vi "Intensity Check.vi"() -> ()   [LabVIEW 2020]
uses:
  <vilib>/Instr/_visa.llb/VISA Configure Serial Port (Instr).vi
panel:
  out "x+1":dbl
  in  "Take signal?":bool
  in  "Step Angle":dbl=10.0 format="%#_13g"
  in  "½Ð¤Å«ö¥ª¤W¨¤ªº°±¤îµ{¦¡":bool
  in  "iXon exposure time (sec)":dbl=0.15
  out "Currently Angle : (Analyzer)  2":string
  out "?":dbl(knob) scale=0.0..360.0
  out "Slide":dbl(slide) scale=400.0..800.0
  in  "Scan mode":bool
  out "1 OK Done":bool
  in  "Axis 1 Move  Angle":dbl=10.0 format="%#_13g"
  in  "Axis 1 High Speed":dbl=50.0
  in  "Axis 2 High Speed":dbl=50.0
  in  "Axis 2":bool
  in  "Axis 1":bool
  in  "Motors VISA resource (COM7)":refnum<visa-resource-name>="COM12"
  out "Seconds  2":dbl
  out "Minutes":dbl
  out "Hours  2":dbl
  out "Wavelength Filter Currently State :":string
  in  "Longest centroid":dbl=700.0
  in  "Sampling range":dbl=5.0
  in  "Shortest centroid":dbl=400.0
  in  "Bandwidth":dbl=10.0
  in  "Wavelength Filter VISA resource":refnum<visa-resource-name>="COM6"
  # "Wavelength"
  # "Motor"
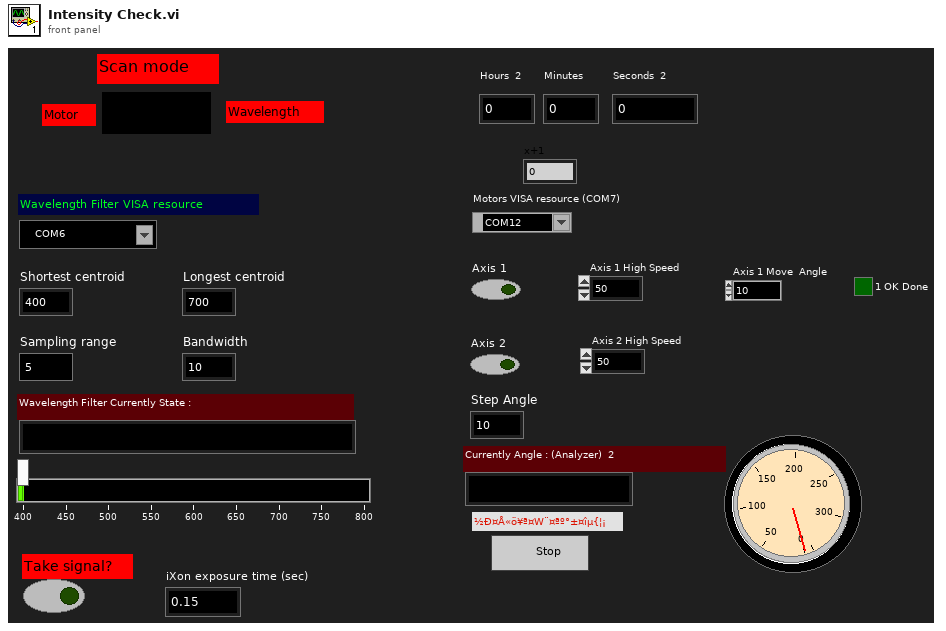
[diagram p1: front panel]
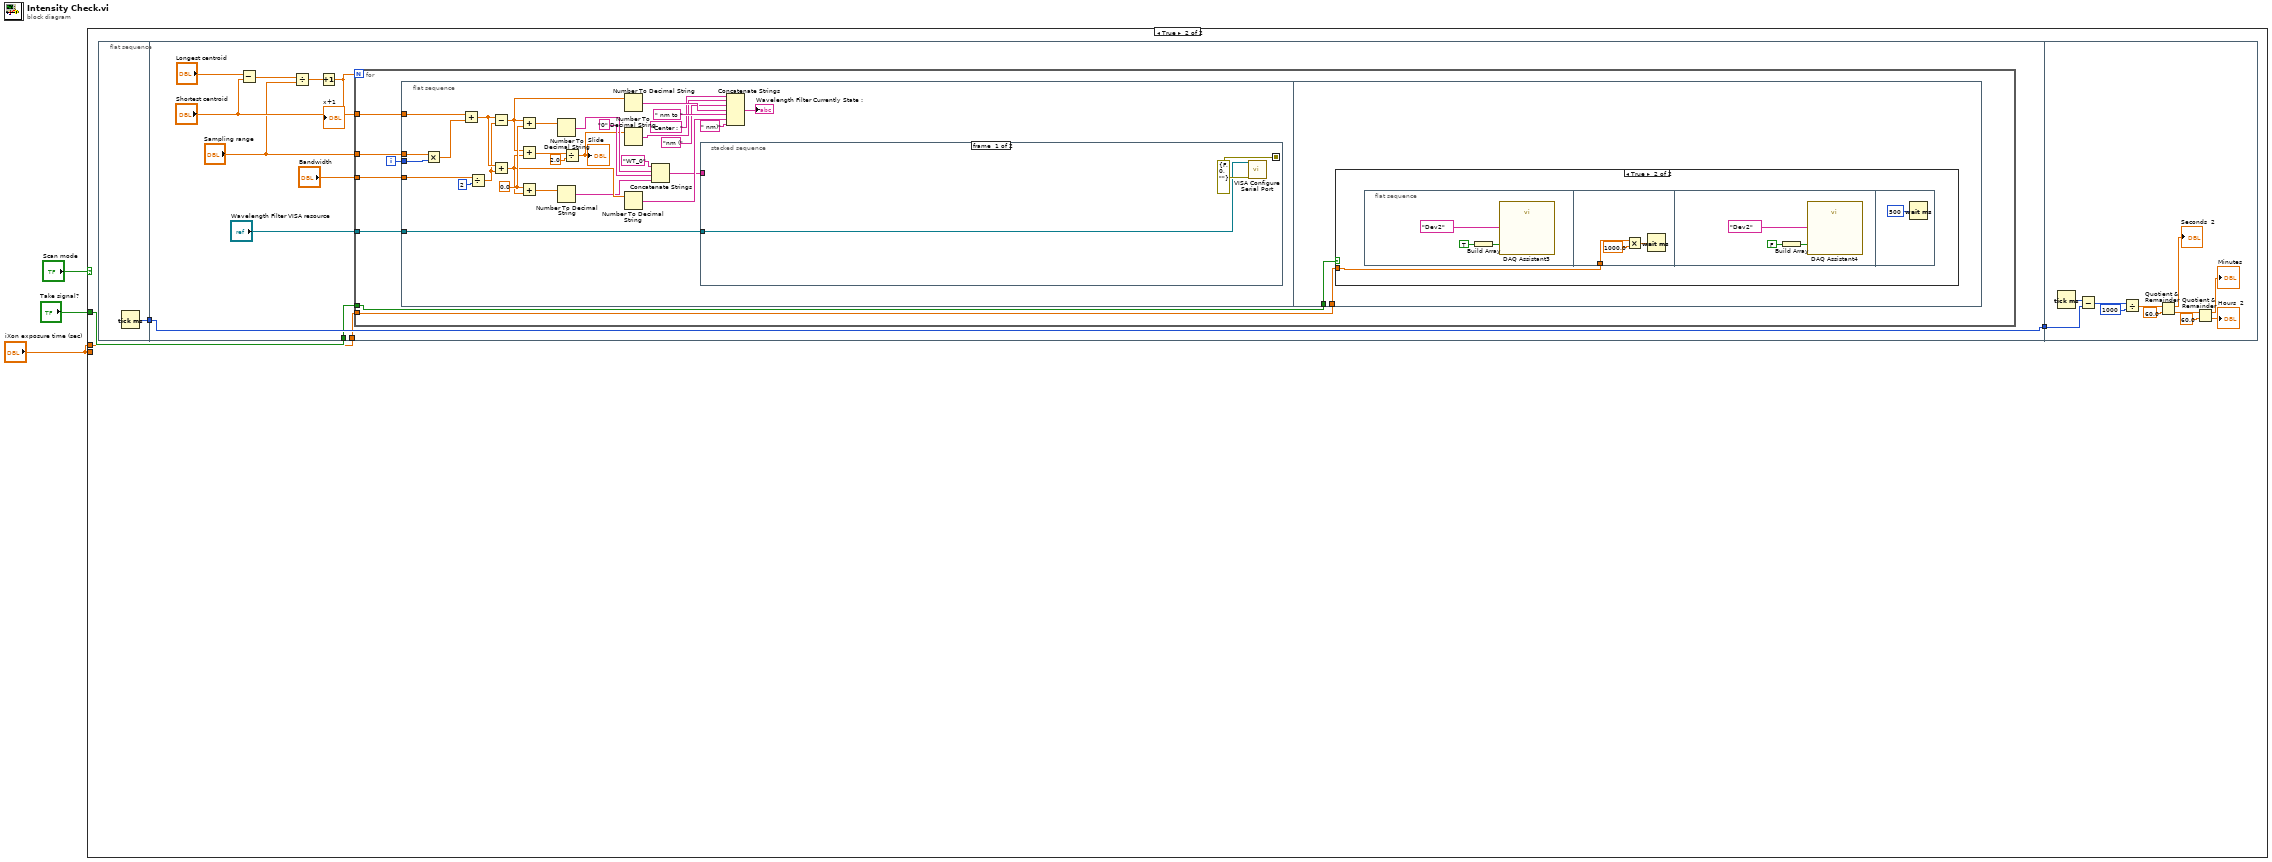
[diagram p0: block diagram]
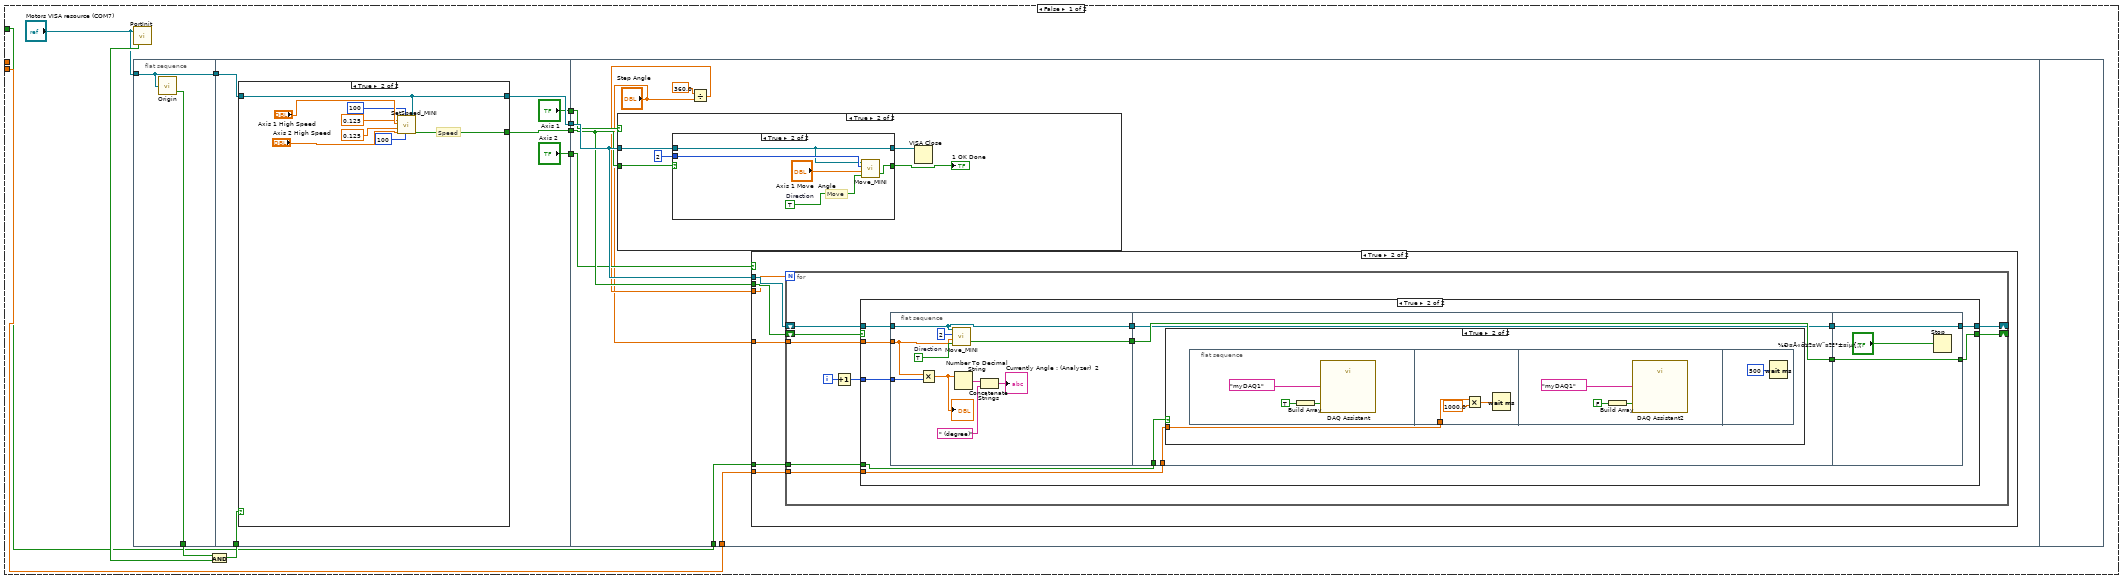
[diagram p2: hidden frame]
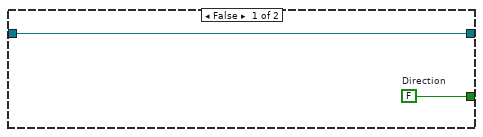
[diagram p3: hidden frame]
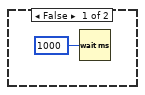
[diagram p6: hidden frame]
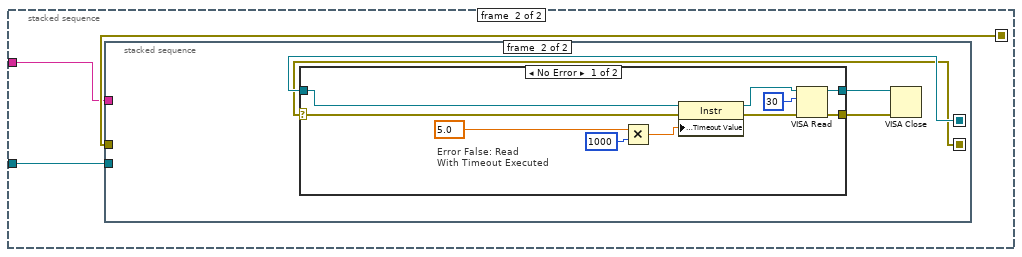
[diagram p9: hidden frame]
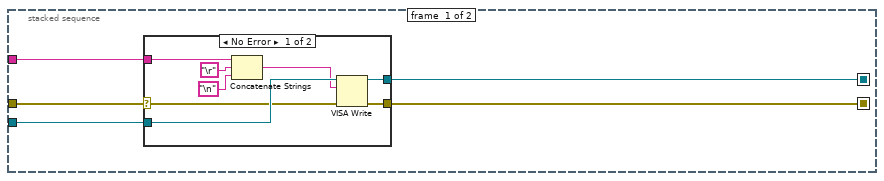
[diagram p10: hidden frame]
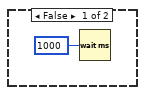
[diagram p13: hidden frame]
diagram:
  n1 = case shown="True" "Scan mode" {
    tunnel: "Take signal?" -> [w4 w112]
    tunnel: "iXon exposure time (sec)" -> [_ w111]
    tunnel: "iXon exposure time (sec)" -> [w5 _]
    frame False {
      n2 = call "PortInit.vi"("VISAリソース名"="Motors VISA resource (COM7)") -> ("Done"=w8:bool)  [unwired: 1 out]
      n3 = flat-sequence {
        tunnel: "Motors VISA resource (COM7)" -> [w16]
        tunnel: [w15] -> w9
        tunnel: [w16] -> w14
        tunnel: w14 -> [w19]
        tunnel: w7 -> [w22]
        tunnel: [w20] -> w12
        tunnel: [w21] -> w13
        tunnel: ["Axis 1"] -> w11
        tunnel: ["Axis 2"] -> w10
        tunnel: w13 -> [w40]
        tunnel: w12 -> [w41]
        tunnel: w11 -> [w39]
        tunnel: w10 -> [w38]
        tunnel: w5 -> [w34]
        tunnel: w4 -> [w33]
        frame #0 {
          n4 = call "Origin.vi"("VISAリソース名"=w16) -> ("OK Done"=w15:bool)  [unwired: 2 out]
        }
        frame #1 {
          n5 = case shown="True" w22 {
            tunnel: [w24 w32] -> w21
            tunnel: w19 -> [w23 w25]
            tunnel: [w23 w25] -> w20
            frame False {
              w24 = FALSE  # Direction
            }
            frame True {
              # "Speed"
              n6 = call "SetSpeed_MINI.vi"("VISAリソース名"=w25, "Acceleration Time2(ms)"=u32 100 ("Acceleration Time 2"), "Acceleration Time1(ms)"=u32 100 ("Acceleration Time 1"), "High Speed2(degrees/s)"="Axis 2 High Speed", "Low Speed2(degrees/s)"=0.125 ("Axis 2 Low Speed"), "High Speed1(degrees/s)"="Axis 1 High Speed", "Low Speed1(degrees/s)"=0.125 ("Axis 1 Low Speed")) -> ("OK Done"=w32:bool)  [unwired: 2 out]
            }
          }
        }
        frame #2 {
          n7 = case shown="True" w39 {
            tunnel: w41 -> [_ w100]
            tunnel: w40 -> [_ w99]
            frame False {
            }
            frame True {
              n8 = case shown="True" w99 {
                selector: w99 -> [w105 _]
                tunnel: [w105 w109] -> w102
                tunnel: 2 ("AxisNumber") -> [_ w110]
                tunnel: w100 -> [w104 w108]
                tunnel: [w104 w108] -> w103
                frame False {
                }
                frame True {
                  w107 = TRUE  # Direction
                  # "Move"
                  n9 = call "Move_MINI.vi"("Direction"=w107, "Step Angle(degree)"="Axis 1 Move  Angle", "Axis Number"=w110, "VISAリソース名"=w108) -> ("OK Done"=w109:bool)  [unwired: 1 in]
                }
              }
              "1 OK Done" <- w102
              n10 = VISA Close(VISA resource name=w103) -> ()  [unwired: 1 in, 1 out]
            }
          }
          n11 = Divide(x=360.0 ("y"), y="Step Angle") -> (x/y=w36:dbl)
          n12 = case shown="True" w38 {
            tunnel: w41 -> [_ w46]
            tunnel: w40 -> [_ w47]
            tunnel: w36 -> [_ w45]
            tunnel: "Step Angle" -> [_ w44]
            tunnel: w34 -> [_ w43]
            tunnel: w33 -> [_ w42]
            frame False {
            }
            frame True {
              n13 = for {
                N: w45 -> [_]
                shift-right: [w52] -> _
                shift-left: w47 -> [w56]
                shift-right: [w53] -> _
                shift-left: w46 -> [w55]
                tunnel: w44 -> [w50]
                tunnel: w43 -> [w49]
                tunnel: w42 -> [w48]
                i -> [w54]
                n14 = Increment(x=w54) -> (x+1=w51:i32)
                n15 = case shown="True" w56 {
                  selector: w56 -> [w58 _]
                  tunnel: [w58 w68] -> w52
                  tunnel: w55 -> [w57 w69]
                  tunnel: [w57 w67] -> w53
                  tunnel: w51 -> [_ w66]
                  tunnel: w50 -> [_ w65]
                  tunnel: w49 -> [_ w60]
                  tunnel: w48 -> [_ w59]
                  frame False {
                  }
                  frame True {
                    n16 = flat-sequence {
                      tunnel: w69 -> [w76]
                      tunnel: [w79] -> w64
                      tunnel: [w76] -> w62
                      tunnel: w66 -> [w73]
                      tunnel: w65 -> [w70]
                      tunnel: w64 -> [w83]
                      tunnel: [w83] -> w63
                      tunnel: w62 -> [w82]
                      tunnel: [w82] -> w61
                      tunnel: w60 -> [w81]
                      tunnel: w59 -> [w80]
                      tunnel: [w98] -> w68
                      tunnel: [w97] -> w67
                      tunnel: w63 -> [w98]
                      tunnel: w61 -> [w97]
                      frame #0 {
                        w78 = TRUE  # Direction
                        n17 = Multiply(x=w70, y=w73) -> (x*y=w71:dbl)
                        "?" <- w71
                        n18 = call "Move_MINI.vi"("Direction"=w78, "Step Angle(degree)"=w70, "Axis Number"=2 ("AxisNumber"), "VISAリソース名"=w76) -> ("OK Done"=w79:bool)  [unwired: 1 in]
                        n19 = Number To Decimal String(number=w71) -> (decimal integer string=w74:string)  [unwired: 1 in]
                        n20 = Concatenate Strings(w74, " (degree)" ("string")) -> (→"Currently Angle : (Analyzer)  2":string)
                      }
                      frame #1 {
                        n21 = case shown="True" w80 {
                          tunnel: w81 -> [_ w85]
                          frame False {
                            n22 = Wait (ms)(milliseconds to wait=u32 1000) -> ()  [unwired: 1 out]
                          }
                          frame True {
                            n23 = flat-sequence {
                              tunnel: w85 -> [w89]
                              frame #0 {
                                n24 = Build Array(TRUE) -> (w88:bool[])
                                n25 = call "DAQ Assistant"("data"=w88, "device name"=tag "myDAQ1") -> ()  [unwired: 16 in, 2 out]
                              }
                              frame #1 {
                                n26 = Multiply(x=w89, y=1000.0) -> (x*y=w91:dbl)
                                n27 = Wait (ms)(milliseconds to wait=w91) -> ()  [unwired: 1 out]
                              }
                              frame #2 {
                                n28 = Build Array(FALSE) -> (w94:bool[])
                                n29 = call "DAQ Assistant2"("data"=w94, "device name"=tag "myDAQ1") -> ()  [unwired: 16 in, 2 out]
                              }
                              frame #3 {
                                n30 = Wait (ms)(milliseconds to wait=u32 500) -> ()  [unwired: 1 out]
                              }
                            }
                          }
                        }
                      }
                      frame #2 {
                        n31 = Stop(stop? (T)="½Ð¤Å«ö¥ª¤W¨¤ªº°±¤îµ{¦¡") -> ()
                      }
                    }
                  }
                }
              }
            }
          }
        }
        frame #3 {
        }
      }
      n32 = Compound Arithmetic op=AND(w9, w8) -> (w7:bool)
    }
    frame True {
      n33 = flat-sequence {
        tunnel: [w115] -> w114
        tunnel: [w119] -> w113
        tunnel: w114 -> [w119]
        tunnel: w112 -> [w117]
        tunnel: w111 -> [w116]
        tunnel: w113 -> [w214]
        frame #0 {
          n34 = Tick Count (ms)() -> (millisecond timer value=w115:u32)
        }
        frame #1 {
          n35 = Subtract(x="Longest centroid", y="Shortest centroid") -> (x-y=w125:dbl)
          n36 = Divide(x=w125, y="Sampling range") -> (x/y=w121:dbl)
          n37 = Increment(x=w121) -> (x+1=w118:dbl)
          "x+1" <- w118
          n38 = for {
            N: w118 -> [_]
            tunnel: "Shortest centroid" -> [w132]
            tunnel: "Sampling range" -> [w131]
            tunnel: "Bandwidth" -> [w130]
            tunnel: "Wavelength Filter VISA resource" -> [w129]
            tunnel: w117 -> [w128]
            tunnel: w116 -> [w127]
            i -> [w133]
            n39 = flat-sequence {
              tunnel: w133 -> [w149]
              tunnel: w132 -> [w155]
              tunnel: w131 -> [w154]
              tunnel: w130 -> [w153]
              tunnel: w129 -> [w142]
              tunnel: w128 -> [w201]
              tunnel: w127 -> [w200]
              frame #0 {
                w141 = 0.0 ("y")
                n40 = Multiply(x=w154, y=w149) -> (x*y=w152:dbl)
                n41 = Add(x=w155, y=w152) -> (x+y=w151:dbl)
                n42 = Divide(x=w153, y=2) -> (x/y=w150:dbl)
                n43 = Subtract(x=w151, y=w150) -> (x-y=w140:dbl)
                n44 = Add(x=w151, y=w150) -> (x+y=w137:dbl)
                n45 = Add(x=w140, y=w141) -> (x+y=w139:dbl)
                n46 = Add(x=w140, y=w137) -> (x+y=w147:dbl)
                n47 = Add(x=w141, y=w137) -> (x+y=w136:dbl)
                n48 = Number To Decimal String(number=w139) -> (decimal integer string=w138:string)  [unwired: 1 in]
                n49 = Number To Decimal String(number=w136) -> (decimal integer string=w135:string)  [unwired: 1 in]
                n50 = Divide(x=w147, y=2.0) -> (x/y=w134:dbl)
                "Slide" <- w134
                n51 = Number To Decimal String(number=w140) -> (decimal integer string=w158:string)  [unwired: 1 in]
                n52 = Number To Decimal String(number=w134) -> (decimal integer string=w145:string)  [unwired: 1 in]
                n53 = Number To Decimal String(number=w137) -> (decimal integer string=w157:string)  [unwired: 1 in]
                n54 = Concatenate Strings("WT_0", w138, "0", w135) -> (w156:string)
                n55 = stacked-sequence {
                  seq-local: [w165 _] -> [_ w168]
                  tunnel: w142 -> [w164 w167]
                  tunnel: w156 -> [_ w166]
                  frame #0 {
                    w165 = errorcluster {"status"=FALSE, "code"=0, "source"=""} ("Error In (no error)")
                    n56 = call-poly "VISA Configure Serial Port"("VISA resource name"=w164, "error in (no error)"=w165) -> ()  [unwired: 12 in, 2 out]
                  }
                  frame #1 {
                    n57 = stacked-sequence {
                      seq-local: [w171 _] -> [_ w185]
                      seq-local: [w170 _] -> [_ w184]
                      tunnel: w167 -> [w173 _]
                      tunnel: w168 -> [w172 _]
                      tunnel: w166 -> [w169 _]
                      frame #0 {
                        n58 = case shown="No Error" w172 {
                          selector: w172 -> [w180 w182]
                          tunnel: w173 -> [w181 w183]
                          tunnel: [w179 w182] -> w170
                          tunnel: [w178 w183] -> w171
                          tunnel: w169 -> [w174 _]
                          frame No Error {
                            n59 = Concatenate Strings(w174, "\r", "\n") -> (w177:string)
                            n60 = VISA Write(VISA resource name=w181, write buffer=w177, error in (no error)=w180) -> (VISA resource name out=w178:refnum<visa-resource-name>, error out=w179:errorcluster)  [unwired: 1 out]
                          }
                          frame Error {
                          }
                        }
                      }
                      frame #1 {
                        n61 = case shown="No Error" w184 {
                          selector: w184 -> [w191 w199]
                          tunnel: [w188 w199] -> w186
                          tunnel: w185 -> [w192 w198]
                          tunnel: [w189 w198] -> w187
                          frame No Error {
                            # "Error False: Read\nWith Timeout Executed"
                            n62 = Multiply(x=5.0 ("Timeout Limit (s)(10)"), y=1000) -> (x*y=w193:dbl)
                            n63 = property class="Instr"(reference=w192, error in=w191, "General Settings:Timeout Value"=w193) -> (reference out=w197:refnum<visa-resource-name>, error out=w196:errorcluster)
                            n64 = VISA Read(VISA resource name=w197, byte count=30 ("Bytes To Read (30)"), error in (no error)=w196) -> (VISA resource name out=w189:refnum<visa-resource-name>, error out=w188:errorcluster)  [unwired: 2 out]
                          }
                          frame Error {
                          }
                        }
                        n65 = VISA Close(VISA resource name=w187, error in (no error)=w186) -> ()  [unwired: 1 out]
                      }
                    }
                  }
                }
                n66 = Concatenate Strings("Center : " ("string"), w145, "nm (" ("string"), w158, " nm to ", w157, " nm)" ("string")) -> (→"Wavelength Filter Currently State :":string)
              }
              frame #1 {
                n67 = case shown="True" w201 {
                  tunnel: w200 -> [_ w203]
                  frame False {
                    n68 = Wait (ms)(milliseconds to wait=u32 1000) -> ()  [unwired: 1 out]
                  }
                  frame True {
                    n69 = flat-sequence {
                      tunnel: w203 -> [w207]
                      frame #0 {
                        n70 = Build Array(TRUE) -> (w206:bool[])
                        n71 = call "DAQ Assistant3"("data"=w206, "device name"=tag "Dev2") -> ()  [unwired: 16 in, 2 out]
                      }
                      frame #1 {
                        n72 = Multiply(x=w207, y=1000.0) -> (x*y=w209:dbl)
                        n73 = Wait (ms)(milliseconds to wait=w209) -> ()  [unwired: 1 out]
                      }
                      frame #2 {
                        n74 = Build Array(FALSE) -> (w212:bool[])
                        n75 = call "DAQ Assistant4"("data"=w212, "device name"=tag "Dev2") -> ()  [unwired: 16 in, 2 out]
                      }
                      frame #3 {
                        n76 = Wait (ms)(milliseconds to wait=u32 500) -> ()  [unwired: 1 out]
                      }
                    }
                  }
                }
              }
            }
          }
        }
        frame #2 {
          n77 = Tick Count (ms)() -> (millisecond timer value=w221:u32)
          n78 = Subtract(x=w221, y=w214) -> (x-y=w222:u32)
          n79 = Divide(x=w222, y=u32 1000) -> (x/y=w223:dbl)
          n80 = Quotient & Remainder(x=w223, y=60.0) -> (x-y*floor(x/y)=→"Seconds  2":dbl, floor(x/y)=w224:dbl)
          n81 = Quotient & Remainder(x=w224, y=60.0) -> (x-y*floor(x/y)=→"Minutes":dbl, floor(x/y)=→"Hours  2":dbl)
        }
      }
    }
  }
